vi "Delete.vi"(11 "TEMPLATE Msg Output in":refnum<class "TEMPLATE Msg Output.lvclass">) -> ()   [LabVIEW 2020, in "_Template.lvlib" / "Templates.lvlib" / "TEMPLATE jettl Msg.lvlib" / "TEMPLATE Msg Output.lvclass"]
uses:
  TEMPLATE Msg Output.lvclass
  TEMPLATE Msg Output.lvclass/TEMPLATE Msg Output.ctl
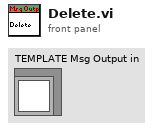
[diagram p1: front panel]
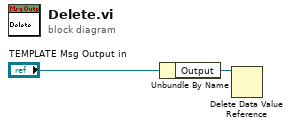
[diagram p0: block diagram]
diagram:
  n1 = Unbundle By Name("TEMPLATE Msg Output in") -> ("Output"=w1:refnum<data-value>)
  n2 = Delete Data Value Reference(data value reference=w1) -> ()  [unwired: 1 in, 2 out]
